vi "Launch DAQMan.vi"   [LabVIEW 2018]
uses:
  Classes/Cfg Grandmaster/Class Cfg Grandmaster/Cfg Grandmaster.lvclass
  C:/Program Files (x86)/National Instruments/LabVIEW 2018/vi.lib/ActorFramework/Actor/Actor.lvclass
  <vilib>/ActorFramework/Message Queue/Message Queue.lvclass/Message Queue.ctl
  <vilib>/ActorFramework/Message Enqueuer/Message Enqueuer.lvclass/Message Enqueuer.ctl
  <vilib>/ActorFramework/Message Enqueuer/Enqueue.vi
  Classes/Cfg Grandmaster/DAQMan Messages/Initialize DAQMan Msg/Initialize DAQMan Msg.lvclass
  C:/Program Files (x86)/National Instruments/LabVIEW 2018/vi.lib/ActorFramework/Message/Message.lvclass
  <vilib>/ActorFramework/Message Priority Queue/Priority Enqueue.vi
  <vilib>/ActorFramework/Actor/Actor.lvclass
  <vilib>/ActorFramework/Message Queue/Message Queue.lvclass
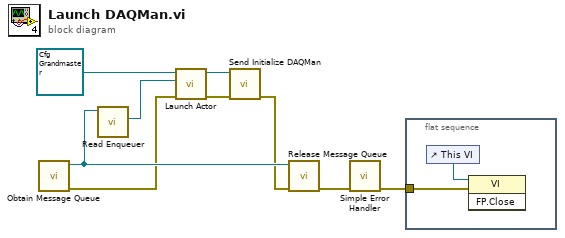
[diagram p0: block diagram]
diagram:
  n1 = call <vilib>:"Obtain Message Queue.vi"() -> ("error out"=w4:errorcluster, "Message Queue"=w8:refnum<class "Message Queue.lvclass">)  [unwired: 10 in]
  n2 = call <vilib>:"Read Enqueuer.vi"("Message Queue"=w8) -> ("Message Enqueuer"=w3:refnum<class "Message Enqueuer.lvclass">)  [unwired: 10 in]
  n3 = call <vilib>:"Launch Actor.vi"("error in (no error)"=w4, "Actor-to-Caller Enqueuer"=w3, "Actor"=refnum<class "Cfg Grandmaster.lvclass"> refnum ("Cfg Grandmaster.lvlib:Cfg Grandmaster.lvclass")) -> ("error out"=w2:errorcluster, "Caller-To-Actor Enqueuer"=w5:refnum<class "Message Enqueuer.lvclass">)  [unwired: 7 in]
  n4 = call "Send Initialize DAQMan.vi"("error in (no error)"=w2, "Message Enqueuer"=w5) -> ("error out"=w1:errorcluster)  [unwired: 8 in, 1 out]
  n5 = call <vilib>:"Release Message Queue.vi"("error in (no error)"=w1, "Message Queue"=w8) -> ("error out"=w7:errorcluster)  [unwired: 8 in, 1 out]
  n6 = call <vilib>:"Simple Error Handler.vi"("error in (no error)"=w7) -> ("error out"=w6:errorcluster)  [unwired: 4 in, 4 out]
  n7 = flat-sequence {
    tunnel: w6 -> [w11]
    frame #0 {
      n8 = control-ref of="This VI"() -> (w10:refnum<vi>)
      n9 = invoke class="VI" method="FP.Close"(reference=w10, error in=w11) -> ()  [unwired: 1 in, 3 out]
    }
  }
